vi "Read_OPC_Product_Date.vi"(1 "Shift":u16, 2 "Date":u16, 3 "Month":u16, 4 "Year":u16) -> (0 "ProductDate":string)   [LabVIEW 2017]
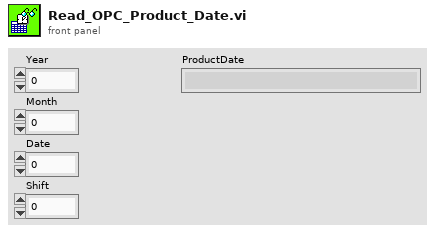
[diagram p1: front panel]
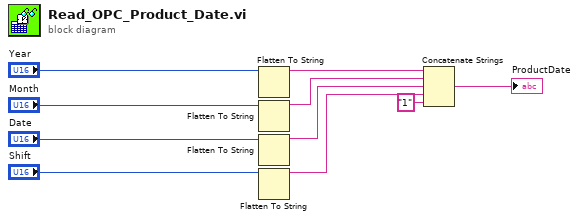
[diagram p0: block diagram]
diagram:
  n1 = Flatten To String(anything="Year") -> (data string=w10:string)  [unwired: 3 in, 2 out]
  n2 = Flatten To String(anything="Month") -> (data string=w9:string)  [unwired: 3 in, 2 out]
  n3 = Flatten To String(anything="Date") -> (data string=w8:string)  [unwired: 3 in, 2 out]
  n4 = Flatten To String(anything="Shift") -> (data string=w7:string)  [unwired: 3 in, 2 out]
  n5 = Concatenate Strings(w10, w9, w8, w7, "1" ("string")) -> (→"ProductDate":string)
